vi "Get DataTable Reft.vi"(8 "error in (no error)":errorcluster caption="错误输入（无错误）", 11 "DataTable输入":refnum<class "DataTable.lvclass">) -> (0 "error out":errorcluster caption="错误输出", 2 "DataTable":refnum<k24>, 3 "DataTable输出":refnum<class "DataTable.lvclass">)   [LabVIEW 2012, in "Data Grid VIEW.lvlib" / "DataTable.lvclass"]
uses:
  DataTable.lvclass
  System.Data
  DataTable.lvclass/DataTable.ctl
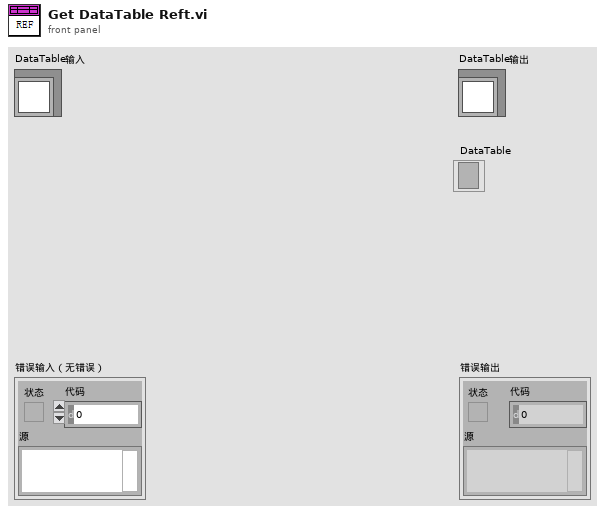
[diagram p1: front panel]
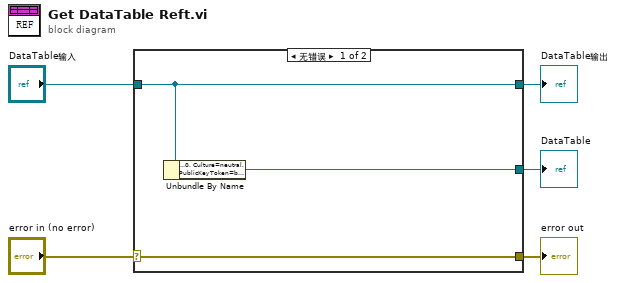
[diagram p0: block diagram]
diagram:
  n1 = case shown="无错误" "error in (no error)" {
    selector: "error in (no error)" -> [w8 w9]
    tunnel: [w8 w9] -> w4
    tunnel: [w7 w10] -> w2
    tunnel: "DataTable输入" -> [w7 w10]
    tunnel: [w6 _] -> w1
    frame No Error {
      n2 = Unbundle By Name(w7) -> ("DataTable"=w6:refnum<k24>)
    }
    frame Error {
    }
  }
  "error out" <- w4
  "DataTable输出" <- w2
  "DataTable" <- w1
